vi "Set Sys objects.vi"(8 "error in (no error)":errorcluster, 10 "System objects":refnum<class "system object.lvclass">[](array[class]), 11 "Folder in":refnum<class "Folder.lvclass">) -> (0 "error out":errorcluster, 3 "Folder out":refnum<class "Folder.lvclass">)   [LabVIEW 2020, in "Folder.lvclass"]
uses:
  Folder.lvclass
  Folder.lvclass/Folder.ctl
  system object/system object.lvclass
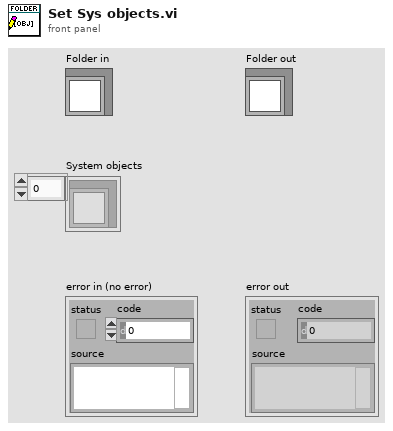
[diagram p1: front panel]
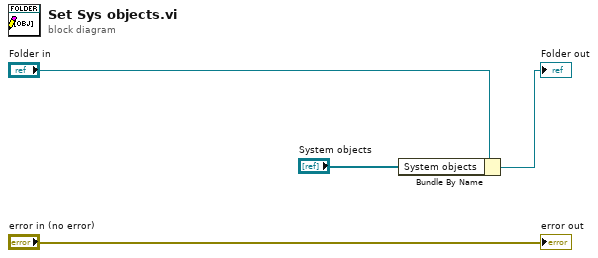
[diagram p0: block diagram]
diagram:
  n1 = Bundle By Name(cluster="Folder in", "System objects"="System objects") -> (→"Folder out":refnum<class "Folder.lvclass">)
  "error out" <- "error in (no error)"
